vi "Real Matrix Exp.vi"(3 "Input Matrix":T1) -> (0 "error":i32, 1 "Matrix Exp":T1)   [LabVIEW 2014, in "NI_AALBase.lvlib"]
doc: "Computes the exponential of a square <B>Input Matrix</B>. Wire data to the <B>Input Matrix</B> input to determine the polymorphic instance to use or manually select the instance."
uses:
  NI_AALBase.lvlib
  RealMatrix.ctl
  lvanlys.dll
  NI_Matrix.lvlib
panel:
  # "Matrix Exp"
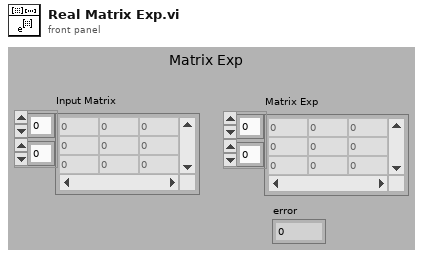
[diagram p1: front panel]
types:
  T1 = typedef "NI_Matrix.lvlib/RealMatrix.ctl" = dbl[][]
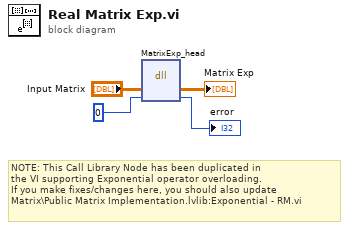
[diagram p0: block diagram]
diagram:
  # "NOTE: This Call Library Node has been duplicated in\nthe VI supporting Exponential operator overloading.\nIf you make fixes/changes here, you should also update\nMatrix\\Public Matrix Implementation.lvlib:Exponential - RM.vi"
  n1 = dll-call lib="C:/Program Files (x86)/National Instruments/LabVIEW 2014/resource/lvanlys.*" fn="MatrixExp_head"("Input Matrix"="Input Matrix", 0) -> ("Input Matrix"=→"Matrix Exp":T1, →"error":i32)  [unwired: 4 in, 2 out]
